vi "Complex Magnitude Square (SGL).vi"(8 "Input Valid":bool=TRUE, 11 "X1+j Y1":cluster{"Y1":fxp<+,32,32>, "X1":fxp<+,32,32>}) -> (0 "Output Valid":bool, 3 "Magnitude Square":fxp<+,32,32>)   [LabVIEW 2012]
doc: "This VI performs single precision complex add\n\n<b> Latency = 11 Ticks </b>"
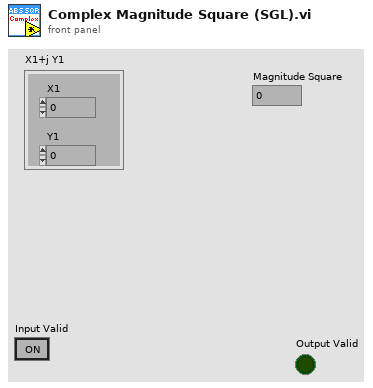
[diagram p1: front panel]
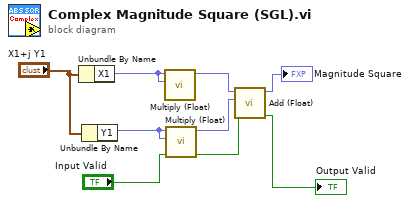
[diagram p0: block diagram]
diagram:
  n1 = Unbundle By Name("X1+j Y1") -> ("X1"=w9:fxp<+,32,32>)
  n2 = Unbundle By Name("X1+j Y1") -> ("Y1"=w7:fxp<+,32,32>)
  n3 = call <userlib>:"Multiply (Float).vi"("b"=w9, "a"=w9) -> ("a*b"=w5:fxp<+,32,32>)  [unwired: 8 in, 1 out]
  n4 = call <userlib>:"Multiply (Float).vi"("Input Valid"="Input Valid", "b"=w7, "a"=w7) -> ("Output Valid"=w3:bool, "a*b"=w4:fxp<+,32,32>)  [unwired: 7 in]
  n5 = call <userlib>:"Add (Float).vi"("Input Valid"=w3, "b"=w4, "a"=w5) -> ("Output Valid"=→"Output Valid":bool, "a+b"=→"Magnitude Square":fxp<+,32,32>)  [unwired: 7 in]
